vi "AsyncTest.vi"() -> ()   [LabVIEW 2015, in "ResultProcessor Tests.lvlib"]
uses:
  ResultProcessor Tests.lvlib
  Execution/ResultProcessor.lvclass
  Config/ResultProcessor Config.lvclass
panel:
  out "AsyncWorkerError":errorcluster
  out "error out":errorcluster
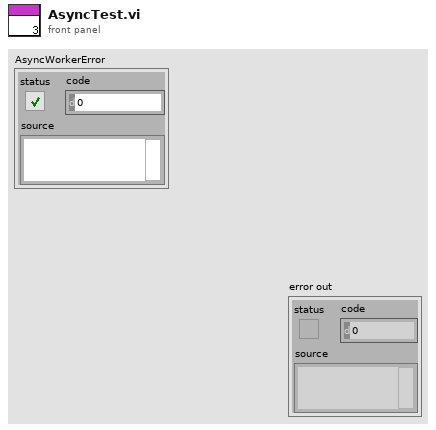
[diagram p1: front panel]
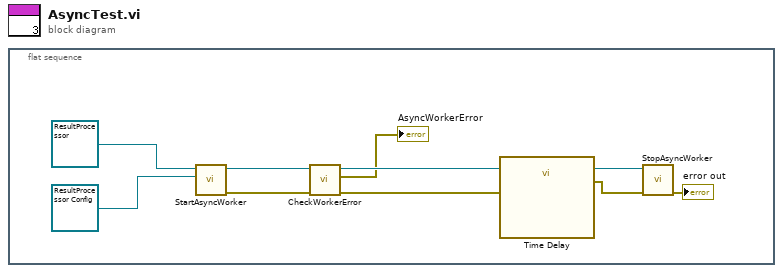
[diagram p0: block diagram]
diagram:
  n1 = flat-sequence {
    frame #0 {
      n2 = call "StartAsyncWorker.vi"("ResultProcessor Config.lvclass"=refnum<class "ResultProcessor Config.lvclass"> refnum, "ResultProcessor in"=refnum<class "ResultProcessor.lvclass"> refnum ("ResultProcessor.lvclass")) -> ("error out"=w2:errorcluster, "ResultProcessor out"=w8:refnum<class "ResultProcessor.lvclass">)  [unwired: 8 in]
      n3 = call "CheckWorkerError.vi"("error in (no error)"=w2, "ResultProcessor in"=w8) -> ("error out"=w4:errorcluster, "AsyncWorkerError"=→"AsyncWorkerError":errorcluster, "ResultProcessor out"=w5:refnum<class "ResultProcessor.lvclass">)  [unwired: 7 in]
      n4 = call "Time Delay"("error in (no error)"=w4) -> ("error out"=w7:errorcluster)  [unwired: 10 in]
      n5 = call "StopAsyncWorker.vi"("error in (no error)"=w7, "ResultProcessor in"=w5) -> ("error out"=→"error out":errorcluster)  [unwired: 8 in, 1 out]
    }
  }
